vi "Actor Core.vi"(8 "error in":errorcluster, 11 "Test Caller Actor in":refnum<class "Test Caller Actor.lvclass">) -> (0 "error out":errorcluster, 3 "Actor out":refnum<class "Actor.lvclass">)   [LabVIEW 2023, in "Test Caller Actor.lvlib" / "Test Caller Actor.lvclass"]
doc: "(<B>Filename</B>: Actor Framework.lvlib:Actor.lvclass:Actor Core.vi)\n\nReceives messages to the actor, reacts to them, and initiates any error handling that may shut the actor down.\n\nDescendant classes may override this VI to append parallel tasks for the actor to complete while it handles messages. Overrides use the Call Parent Class Method node."
uses:
  Test Caller Actor.lvclass
  <vilib>/ActorFramework/Actor/Actor.lvclass
  Abstract Class/Abstract Class.lvclass
  Test Caller Actor.lvclass/Test Caller Actor.ctl
  <vilib>/ActorFramework/Stop Msg/Stop Msg.lvclass
  <vilib>/ActorFramework/Message Enqueuer/Message Enqueuer.lvclass
  <userlib>/_OpenG.lib/error/error.llb/openg_error.lvlib
  Class Loader/Class Loader Messages/Load Msg/Load Msg.lvclass
  <userlib>/_OpenG.lib/time/time.llb/openg_time.lvlib
  Class Loader/Class Loader/Loading Progress.ctl
  Class Loader/Class Loader/Class Loader.lvclass
  Class Loader/Class Loader/Loading Method.ctl
panel:
  out "Timing (s)":dbl
  in  "Loading Method":T1
  in  "Exit":bool
  in  "Load Concrete Classes":bool
  out "Class Names":string[](array[string])
  out "Load Complete":bool
  out "Loading Progress":T2 scale=0.0..100.0
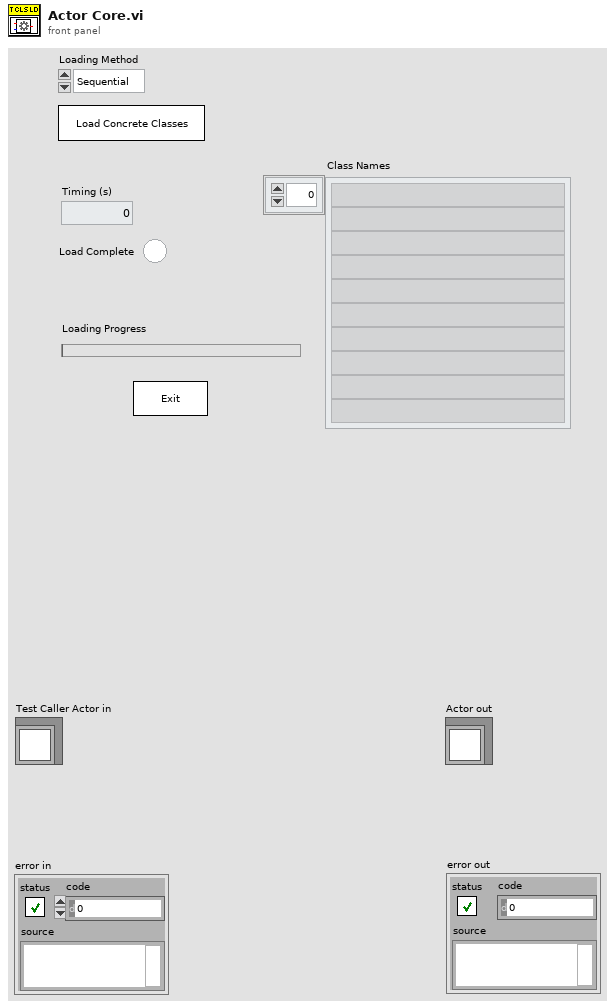
[diagram p1: front panel]
types:
  T1 = typedef "Class Loader.lvlib/Class Loader.lvclass/Loading Method.ctl" = enum16{"Sequential", "Parallel"}
  T2 = typedef "Class Loader.lvlib/Class Loader.lvclass/Loading Progress.ctl" = dbl
  T3 = enum32{"Invalid", "Standard", "Closed", "Hidden", "Minimized", "Maximized"}
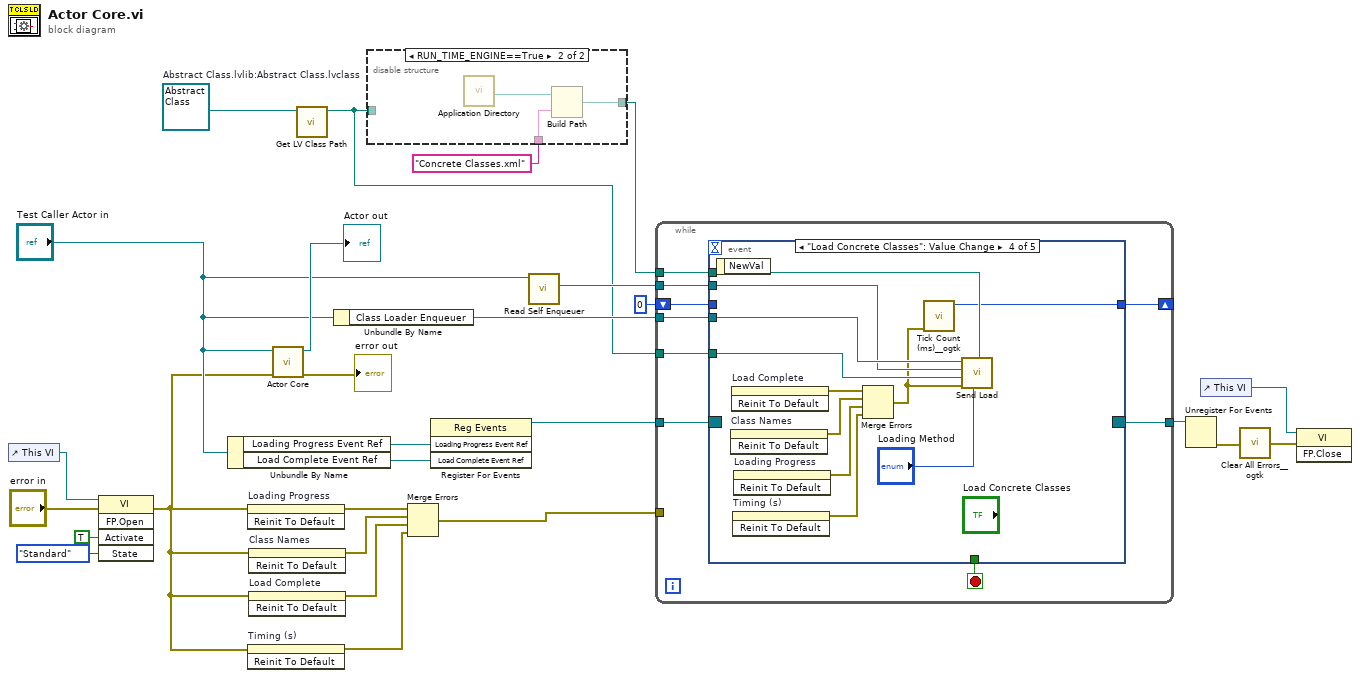
[diagram p0: block diagram]
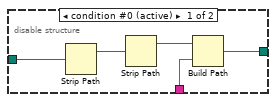
[diagram p2: hidden frame]
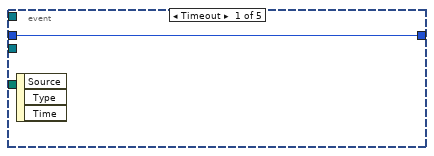
[diagram p3: hidden frame]
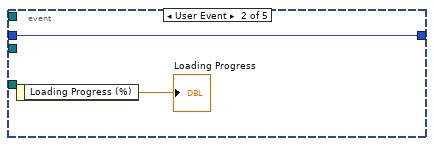
[diagram p4: hidden frame]
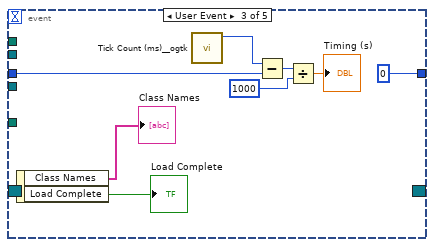
[diagram p5: hidden frame]
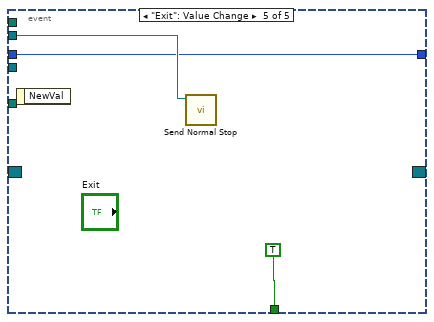
[diagram p6: hidden frame]
diagram:
  w2 = refnum<class "Abstract Class.lvclass"> refnum  # Abstract Class.lvlib:Abstract Class.lvclass
  n1 = control-ref of="This VI"() -> (w13:refnum<vi>)
  n2 = invoke class="VI" method="FP.Open"(reference=w13, error in="error in", "Activate"=TRUE ("Activate?"), "State"=T3."Standard") -> (error out=w5:errorcluster)  [unwired: 1 in, 4 out]
  n3 = Unbundle By Name("Test Caller Actor in") -> ("Loading Progress Event Ref"=w26:refnum<user-event>, "Load Complete Event Ref"=w21:refnum<user-event>)
  n4 = invoke on="Loading Progress" class="Slide (strict)" method="Reinit To Default"(error in=w5) -> (error out=w24:errorcluster)  [unwired: 2 in, 2 out]
  n5 = invoke on="Timing (s)" class="DigNum (strict)" method="Reinit To Default"(error in=w5) -> (error out=w4:errorcluster)  [unwired: 2 in, 2 out]
  n6 = invoke on="Class Names" class="Arr (strict)" method="Reinit To Default"(error in=w5) -> (error out=w19:errorcluster)  [unwired: 2 in, 2 out]
  n7 = invoke on="Load Complete" class="Bool (strict)" method="Reinit To Default"(error in=w5) -> (error out=w18:errorcluster)  [unwired: 2 in, 2 out]
  n8 = call-parent "Actor Core.vi"("error in"=w5, "Actor in"="Test Caller Actor in") -> ("error out"=→"error out":errorcluster, "Actor out"=→"Actor out":refnum<class "Actor.lvclass">)  [unwired: 8 in]
  n9 = call <vilib>:"Get LV Class Path.vi"("object"=w2) -> ("class path"=w1:path)  [unwired: 9 in, 1 out]
  n10 = Unbundle By Name("Test Caller Actor in") -> ("Class Loader Enqueuer"=w6:refnum<class "Message Enqueuer.lvclass">)
  n11 = disable-structure shown="RUN_TIME_ENGINE==True" {
    disable-tunnel: "Concrete Classes.xml" -> [w30 w35]
    disable-tunnel: [w29 w34] -> w15
    disable-tunnel: w1 -> [w28 _]
    frame condition #0 (active) {
      n12 = Strip Path(path=w28) -> (stripped path=w32:path)  [unwired: 1 out]
      n13 = Strip Path(path=w32) -> (stripped path=w31:path)  [unwired: 1 out]
      n14 = Build Path(base path=w31, name or relative path=w30) -> (appended path=w29:path)
    }
    frame condition #1 {
      n15 = call <vilib>:"Application Directory.vi"() -> ("Application Directory"=w33:path)
      n16 = Build Path(base path=w33, name or relative path=w35) -> (appended path=w34:path)
    }
  }
  n17 = Merge Errors(w24, w19, w18, w4) -> (w20:errorcluster)
  n18 = register-events(w26, w21) -> (reference out=w25:refnum<event-registration>)  [unwired: 2 in, 1 out]
  n19 = call <vilib>:"Read Self Enqueuer.vi"("Actor"="Test Caller Actor in") -> ("Self Enqueuer"=w14:refnum<class "Message Enqueuer.lvclass">)  [unwired: 10 in]
  n20 = while {
    tunnel: w25 -> [w44]
    tunnel: w20 -> [_]
    tunnel: [w42] -> w23
    tunnel: w6 -> [w41]
    tunnel: w14 -> [w40]
    tunnel: w15 -> [w39]
    tunnel: w1 -> [w38]
    shift-right: [w37] -> _
    shift-left: u32 0 ("millisecond timer value") -> [w36]
    stop <- w43 stop-if-true
    n21 = event shown="[3] \"Load Concrete Classes\": Value Change" {
      selector: w44 -> [_ _ _ _ _]
      dyn-events: [_ _ _ _ _] -> w42
      timeout: _ -> [_ _ _ _ _]
      tunnel: [_ _ _ _ TRUE ("Exit")] -> w43
      tunnel: w41 -> [_ _ _ w63 _]
      tunnel: w40 -> [_ _ _ w62 w69]
      tunnel: w39 -> [_ _ _ w61 _]
      tunnel: w38 -> [_ _ _ w60 _]
      tunnel: [w45 w46 u32 0 ("millisecond timer value") w56 w67] -> w37
      tunnel: w36 -> [w45 w46 w48 _ w67]
      event Timeout {
        n22 = event-data() -> ()  [unwired: 1 in, 3 out]
      }
      event User Event {
        n23 = event-data() -> ("Loading Progress (%)"=→"Loading Progress":T2)  [unwired: 1 in]
      }
      event User Event {
        n24 = event-data() -> ("Class Names"=→"Class Names":string[], "Load Complete"=→"Load Complete":bool)  [unwired: 1 in]
        n25 = call <userlib>:"Tick Count (ms)__ogtk.vi"() -> ("millisecond timer value"=w49:u32)  [unwired: 10 in, 1 out]
        n26 = Subtract(x=w49, y=w48) -> (x-y=w53:u32)
        n27 = Divide(x=w53, y=u32 1000) -> (x/y=→"Timing (s)":dbl)
      }
      event "Load Concrete Classes": Value Change {
        n28 = event-data() -> ()  [unwired: 1 in, 1 out]
        n29 = invoke on="Class Names" class="Arr (strict)" method="Reinit To Default"() -> (error out=w65:errorcluster)  [unwired: 3 in, 2 out]
        n30 = invoke on="Load Complete" class="Bool (strict)" method="Reinit To Default"() -> (error out=w66:errorcluster)  [unwired: 3 in, 2 out]
        n31 = invoke on="Timing (s)" class="DigNum (strict)" method="Reinit To Default"() -> (error out=w58:errorcluster)  [unwired: 3 in, 2 out]
        n32 = invoke on="Loading Progress" class="Slide (strict)" method="Reinit To Default"() -> (error out=w64:errorcluster)  [unwired: 3 in, 2 out]
        n33 = Merge Errors(w66, w65, w64, w58) -> (w57:errorcluster)
        n34 = call <userlib>:"Tick Count (ms)__ogtk.vi"("error in (no error)"=w57) -> ("millisecond timer value"=w56:u32)  [unwired: 9 in, 1 out]
        n35 = call "Send Load.vi"("Class Relative Paths Path"=w61, "Loading Method"="Loading Method", "error in (no error)"=w57, "Reference Class Path"=w60, "Caller Enqueuer"=w62, "Message Enqueuer in"=w63) -> ()  [unwired: 4 in, 2 out]
      }
      event "Exit": Value Change {
        n36 = event-data() -> ()  [unwired: 1 in, 1 out]
        n37 = call <vilib>:"Send Normal Stop.vi"("Message Enqueuer"=w69) -> ()  [unwired: 10 in, 1 out]
      }
    }
  }
  n38 = Unregister For Events(event registration refnum=w23) -> (error out=w22:errorcluster)  [unwired: 1 in]
  n39 = control-ref of="This VI"() -> (w8:refnum<vi>)
  n40 = call <userlib>:"Clear All Errors__ogtk.vi"("Error In"=w22) -> ("Error Out"=w9:errorcluster)  [unwired: 3 in]
  n41 = invoke class="VI" method="FP.Close"(reference=w8, error in=w9) -> ()  [unwired: 1 in, 3 out]
